vi "FromRepo.vi"(8 "error in":errorcluster, 9 "from repo cluster":T2, 10 "repository in":refnum<class "NISE_CEF_Repository.lvclass">, 11 "node in":refnum<class "Pages.lvclass">) -> (0 "error out":errorcluster, 2 "repository out":refnum<class "NISE_CEF_Repository.lvclass">, 3 "node":T1)   [LabVIEW 2015, in "Pages.lvclass"]
doc: "Grabs information from the Repo and stores it in the nodes."
uses:
  Pages.lvclass
  <vilib>/NI/Configuration Framework/Repository/NISE_CEF_Repository.lvclass
  <vilib>/NI/Configuration Framework/Node/FromRepoCluster.ctl
  <vilib>/NI/Configuration Framework/Node/NodeRef.ctl
  <vilib>/NI/Configuration Framework/Node/NISE_CEF_Node.lvclass
  CustomDeviceRepo/CustomDeviceRepo.lvclass
  CustomDeviceRepo/CustomDeviceRepo.lvclass/CustomDeviceRepo.ctl
  Pages.lvclass/Pages.ctl
  CustomDeviceRepo/Read All Pages Properties.vi
  Write Section Name.vi
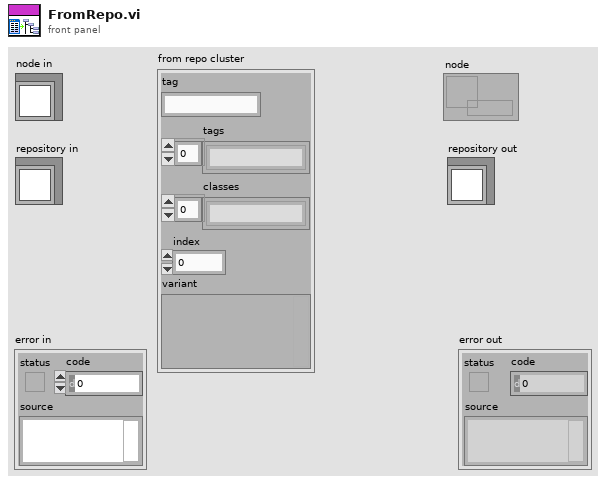
[diagram p1: front panel]
types:
  T1 = typedef "NISE_CEF_Node.lvclass/NodeRef.ctl" = refnum<data-value>
  T2 = typedef "NISE_CEF_Node.lvclass/FromRepoCluster.ctl" = cluster{"tag":string, "tags":string[], "classes":string[], "index":i32, "variant":variant}
  T3 = typedef "Page Properties.ctl" = cluster{"Name":string, "Disallow Renaming":bool, "Delete Protection":bool, "Exlcude from Alphabetical order":bool, "Allow Multi-Selection":bool, "GUID":string, "Parent GUIDs":string[], "Glyph":T4, "Inactive Glyph":T4, "Broken Glyph":T4, "Item to Launch":T4, "Additional Information":string, "Copy":enum16{"copy", "disabled"}, "Paste":enum16{"Create", "CreatIfNotExists_GUID", "CreatIfNotExists_Name", "Replace", "Dialog"}, "Help":T5}
  T4 = typedef "Path Cluster.ctl" = cluster{"Path":path, "Path Type":enum16{"Absolute", "To Base", "To Common Doc Dir", "To Application Data Dir"}}
  T5 = typedef "help.ctl" = cluster{"Item to Launch":T4, "Section":string, "File Type":enum16{"chm", "other"}}
  T6 = typedef "ActionVIs Properties.ctl" = cluster{"Action VI On Delete":T4, "Action VI On Load":T4, "Action VI On Paste":T4, "Action VI On Target Type Change":T4, "Action VI On Delete Request":T4, "Action VI On Compile":T4, "Action VI On System Shutdown":T4, "Action VI On Save":T4, "Action VI On Download":T4}
  T7 = typedef "ButtonLists Properties.ctl" = cluster{"ID":string, "Glyph":T4, "Button Type":T8, "Referenced GUID":string, "Button Text":string, "Caption":string, "Tip Strip":string, "Documentation":string, "Dependency":T9}
  T8 = typedef "Button Type.ctl" = enum16{"Action", "Dialog", "Page", "Notification", "Separator"}
  T9 = typedef "Dependency three item small.ctl" = cluster{"File Path Control":path, "Path Type":enum16{"Absolute", "To Base", "To Common Doc Dir", "To Application Data Dir"}, "Behavior":enum16{"Static", "Dynamic"}}
  T10 = typedef "RunTimeMenus Properties.ctl" = cluster{"GUID":string, "Execution":T11, "MinNrOfChilds":u32, "Name":string, "Item to Launch":T4, "Dependency":T9, "Custom Population":T4, "Menu Item Type":enum16{"Action", "VI", "Separator", "Custom"}, "Behavior":enum16{"Nothing", "Open Front Panel"}, "Position":enum16{"Centered", "Mouse Pointer"}}
  T11 = typedef "Execution Types.ctl" = enum16{"silent", "modal", "floating", "default"}
  T12 = cluster{"General Page Properties":T3, "ActionVIs Properties":T6, "Button List Properties":T7[], "RunTime Menus Properties":T10[]}[]
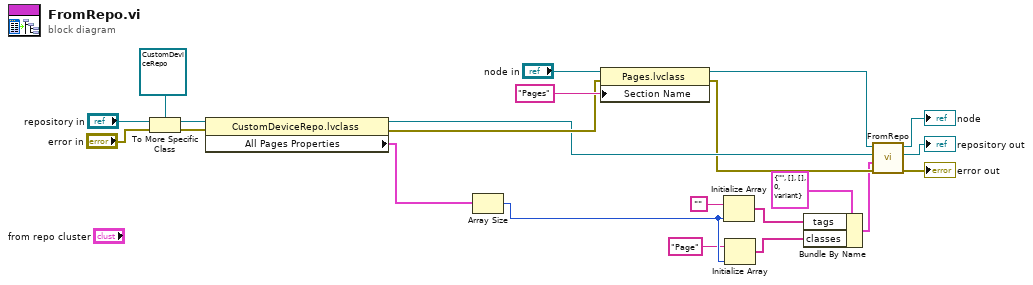
[diagram p0: block diagram]
diagram:
  n1 = To More Specific Class(target class=refnum<class "CustomDeviceRepo.lvclass"> refnum ("CustomDeviceRepo.lvclass"), reference="repository in", error in="error in") -> (specific class reference=w18:refnum<class "CustomDeviceRepo.lvclass">, error out=w19:errorcluster)
  n2 = property class="CustomDeviceRepo.lvclass"(reference=w18, error in=w19) -> (reference out=w11:refnum<class "CustomDeviceRepo.lvclass">, error out=w12:errorcluster, "All Pages Properties"=w8:T12)
  n3 = Array Size(array=w8) -> (size(s)=w6:i32)
  n4 = property class="Pages.lvclass"(reference="node in", error in=w12, "Section Name"="Pages") -> (reference out=w10:refnum<class "Pages.lvclass">, error out=w9:errorcluster)
  n5 = Initialize Array("", w6) -> (w2:string[])
  n6 = Initialize Array("Page", w6) -> (w3:string[])
  n7 = Bundle By Name(cluster=T2 {"tag"="", "tags"=[], "classes"=[], "index"=0, "variant"=variant} ("from repo cluster"), "tags"=w2, "classes"=w3) -> (w1:T2)
  n8 = call-parent "FromRepo.vi"("error in"=w9, "from repo cluster"=w1, "repository in"=w11, "node in"=w10) -> ("error out"=→"error out":errorcluster, "repository out"=→"repository out":refnum<class "NISE_CEF_Repository.lvclass">, "node"=→"node":T1)  [unwired: 5 in]
